vi "Polymerize.vi"(11 "Puzzle In":T1) -> (3 "Puzzle":T1)   [LabVIEW 2020]
uses:
  Puzzle 14.ctl
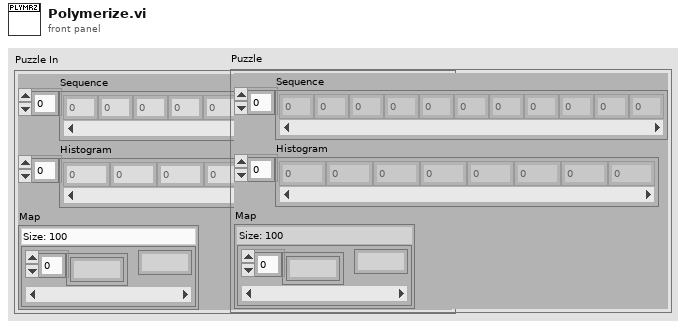
[diagram p1: front panel]
types:
  T1 = typedef "Puzzle 14.ctl" = cluster{"Sequence":u8[], "Histogram":u64[], "Map":map{u8[], u8}}
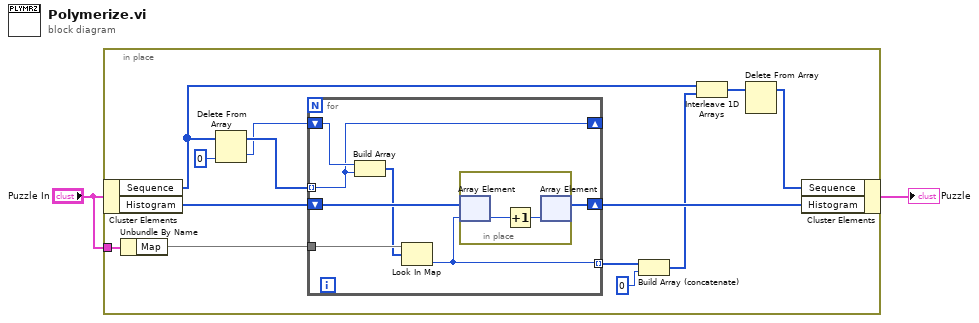
[diagram p0: block diagram]
diagram:
  n1 = in-place {
    in-place-border: "Puzzle In" -> [w15]
    n2 = in-place-cluster #1("Puzzle In") -> ("Sequence"=w7:u8[], "Histogram"=w14:u64[])
    n3 = Unbundle By Name(w15) -> ("Map"=w12:map{u8[], u8})
    n4 = Delete From Array(array=w7, index=0) -> (deleted portion=w9:u8, array with subset deleted=w11:u8[])  [unwired: 1 in]
    n5 = for {
      tunnel: w11 -> [w21] mode=indexing
      shift-right: [w19] -> w13
      shift-left: w14 -> [w20]
      tunnel: w12 -> [w18]
      shift-right: [w21] -> _
      shift-left: w9 -> [w22]
      tunnel: [w17] -> w8 mode=indexing
      n6 = Build Array(w22, w21) -> (w16:u8[])
      n7 = Look In Map(map=w18, key=w16) -> (value=w17:u8)  [unwired: 1 in, 1 out]
      n8 = in-place {
        n9 = in-place-array #2(w20, w17) -> (w24:u64)
        n10 = Increment(x=w24) -> (x+1=w23:u64)
        n11 = in-place-array #2(w23) -> (w19:u64[])  [unwired: 1 out]
      }
    }
    n12 = Build Array (concatenate)(w8, u8 0) -> (w4:u8[])
    n13 = Interleave 1D Arrays(w7, w4) -> (w6:u8[])
    n14 = Delete From Array(array=w6) -> (array with subset deleted=w5:u8[])  [unwired: 2 in, 1 out]
    n15 = in-place-cluster #1("Sequence"=w5, "Histogram"=w13) -> (→"Puzzle":T1)
  }
